vi "CameraSend Images To PC Loop.vi"(8 "error in (no error)":errorcluster, 11 "CameraDevRef":T1) -> ()   [LabVIEW 2014]
doc: "This VI is used to send images to the dashboard using the second enet port on the 8 slot controller. This is provided for compatibility, but is higher overhead than using the Camera MJPG approach.\n\nThis software is licensed. Open the labview\\readme\\WPI Robotics Library Open Source License.txt file for more information."
uses:
  <vilib>/Rock Robotics/WPI/Camera/WPI_CameraDevRef.ctl
  typedefs/vision/vision enable.ctl
  <vilib>/Rock Robotics/SystemInterfaces/NetworkCommunication/NetComm_UsageReport_ResourceType.ctl
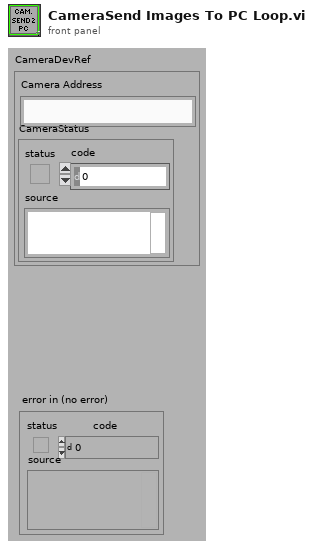
[diagram p1: front panel]
types:
  T1 = typedef "WPI_CameraDevRef.ctl" = cluster{"Camera Address":string, "CameraStatus":errorcluster}
  T2 = typedef "vision enable.ctl" = enum16{"Enable", "Disable", "Stop"}
  T3 = cluster{"fps":i32, "compression":i32, "compression 2":i32}
  T4 = typedef "NetComm_UsageReport_ResourceType.ctl" = enum8{"Controller", "Module", "Language", "CANPlugin", "Accelerometer", "ADXL345", "AnalogChannel", "AnalogTrigger", "AnalogTriggerOutput", "CANJaguar", "Compressor", "Counter", "Dashboard", "DigitalInput", "DigitalOutput", "DriverStationCIO", "DriverStationEIO", "DriverStationLCD", "Encoder", "GearTooth", "Gyro", "I2C", "Framework", "Jaguar", "Joystick", "Kinect", "KinectStick", "PIDController", "Preferences", "PWM", "Relay", "RobotDrive", "SerialPort", "Servo", "Solenoid", "SPI", "Task", "Ultrasonic", "Victor", "Button", "Command", "AxisCamera", "PCVideoServer", "SmartDashboard", "Talon", "HiTechnicColorSensor", "HiTechnicAccel", "HiTechnicCompass", "SRF08", "AnalogOutput", "Victor SP", "Talon SRX", "CAN Talon SRX"}
  T5 = enum16{"Update Mode", "Get Image", "Get Image Data"}
  T6 = typedef "Image Type" = u32
  T7 = typedef "IMAQ Image.ctl" = refnum<image>
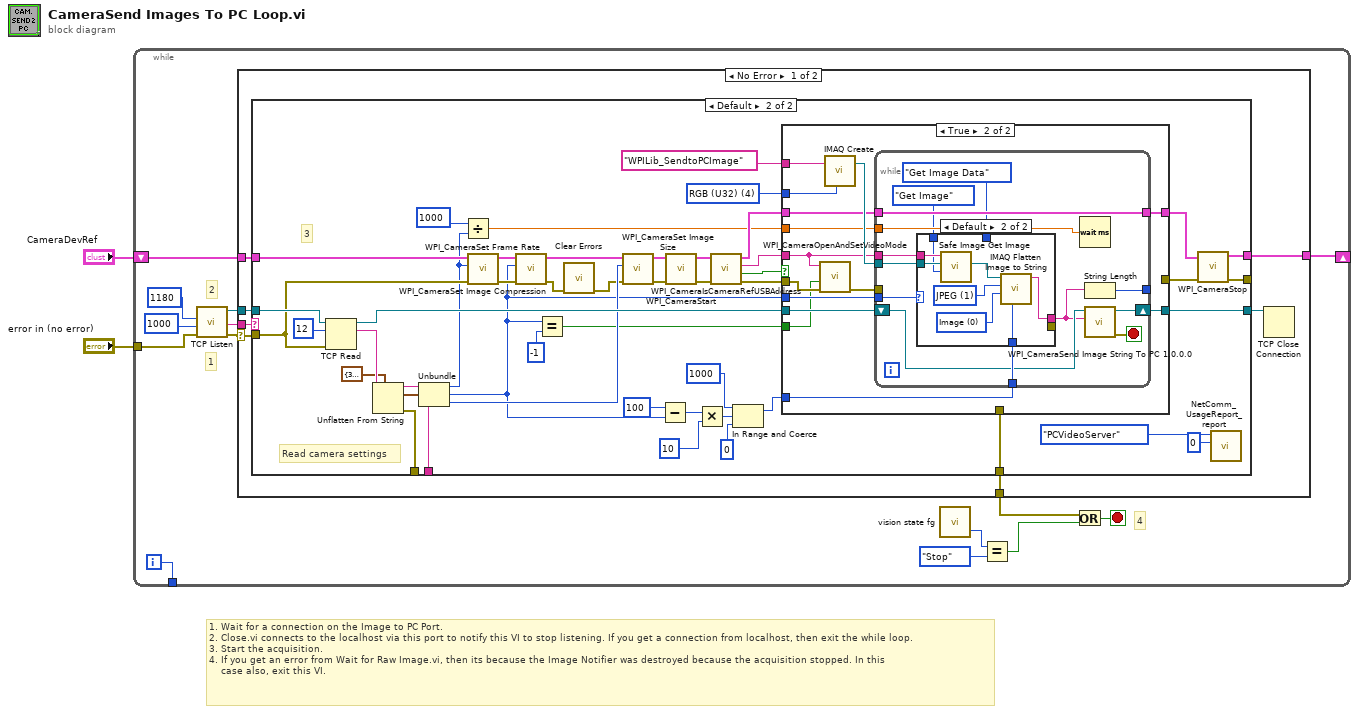
[diagram p0: block diagram]
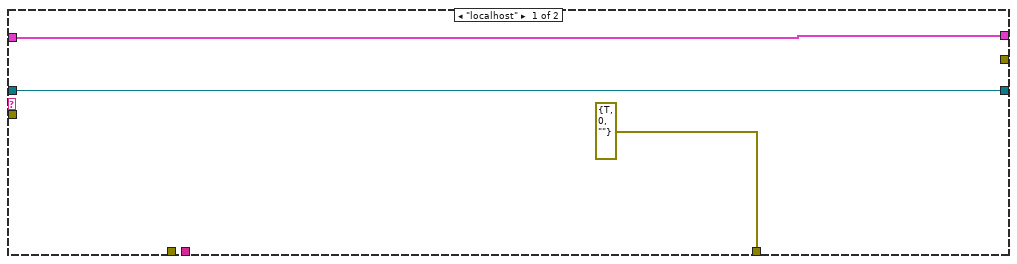
[diagram p2: hidden frame]
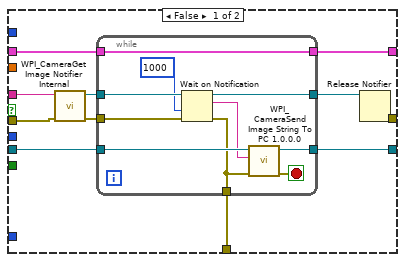
[diagram p3: hidden frame]
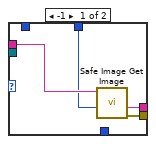
[diagram p4: hidden frame]
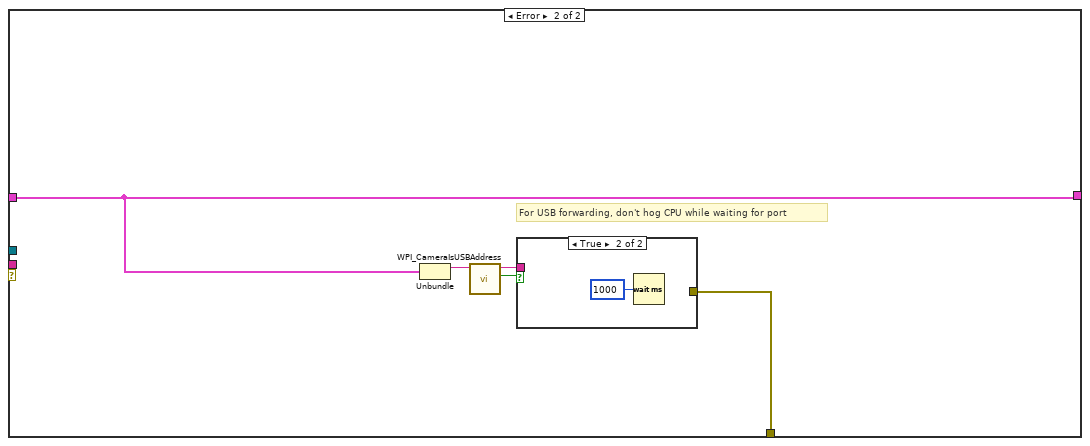
[diagram p5: hidden frame]
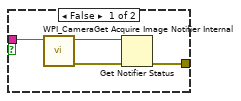
[diagram p6: hidden frame]
diagram:
  # "1. Wait for a connection on the Image to PC Port.\n2. Close.vi connects to the localhost via this port to notify this VI to stop listening. If you get a connection from localhost, then exit the while loop.\n3. Start the acquisition.\n4. If you get an error from Wait for Raw Image.vi, then its because the Image Notifier was destroyed because the acquisition stopped. In this\n    case also, exit this VI."
  n1 = while {
    tunnel: "error in (no error)" -> [w13]
    shift-right: [w16] -> _
    shift-left: "CameraDevRef" -> [w14]
    tunnel: [w8] -> _
    i -> [w8]
    stop <- w5 stop-if-true
    # "4"
    # "1"
    # "2"
    n2 = call <vilib>:"TCP Listen.vi"("error in (no error)"=w13, "timeout ms (wait forever: -1)"=u16 1000 ("port"), "port"=u16 1180) -> ("error out"=w10:errorcluster, "remote address"=w15:string, "connection ID"=w12:refnum<k5>)  [unwired: 1 in, 5 out]
    n3 = case shown="No Error" w10 {
      selector: w10 -> [w17 _]
      tunnel: [w23 w137] -> w16
      tunnel: w15 -> [w22 _]
      tunnel: w14 -> [w21 w137]
      tunnel: w12 -> [w20 _]
      tunnel: [w19 w138] -> w4
      frame No Error {
        n4 = case shown="Default" w22 {
          tunnel: [w26 w71] -> w23
          tunnel: w21 -> [w26 w53]
          tunnel: w17 -> [_ w49]
          tunnel: w20 -> [w24 w57]
          tunnel: [errorcluster {"status"=TRUE, "code"=0, "source"=""} ("error out 2") w73] -> w19
          tunnel: [w24 w72] -> w18
          tunnel: [_ w70] -> _
          tunnel: [_ w28] -> _
          tunnel: [_ w27] -> _
          frame "localhost" {
          }
          frame Default {
            w64 = T6 4 items=["Grayscale (U8)", "Grayscale (I16)", "Grayscale (SGL)", "Complex (CSG)", "RGB (U32)", "HSL (U32)", "RGB (U64)", "Grayscale (U16)"] ("Image Type")
            # "Read camera settings"
            # "3"
            n5 = TCP Read(connection ID=w57, bytes to read=12, error in (no error)=w49) -> (connection ID out=w56:refnum<k5>, data out=w54:string)  [unwired: 2 in, 1 out]
            n6 = Unflatten From String(type=T3 {"fps"=30, "compression"=32, "compression 2"=32} ("Camera Settings"), binary string=w54) -> (rest of the binary string=w27:string, value=w46:T3, error out=w28:errorcluster)  [unwired: 3 in]
            n7 = Unbundle(w46) -> ("fps"=w43:i32, "compression"=w32:i32, "compression 2"=w45:i32)
            n8 = Divide(x=u16 1000 ("port"), y=w43) -> (x/y=w42:dbl)
            n9 = call <vilib>:"WPI_CameraSet Frame Rate.vi"("error in (no error)"=w49, "Frame Rate (fps)"=w43, "CameraDevRef"=w53) -> ("error out"=w48:errorcluster, "CameraDevRef Out"=w52:T1)  [unwired: 7 in]
            n10 = call <vilib>:"WPI_CameraSet Image Compression.vi"("error in (no error)"=w48, "Compression"=w32, "CameraDevRef"=w52) -> ("error out"=w30:errorcluster, "CameraDevRef Out"=w51:T1)  [unwired: 7 in]
            n11 = Equal?(x=w32, y=-1) -> (x = y?=w31:bool)
            n12 = call <vilib>:"Clear Errors.vi"("error in (no error)"=w30) -> ("error out"=w29:errorcluster)  [unwired: 5 in, 1 out]
            n13 = call <vilib>:"WPI_CameraSet Image Size.vi"("error in (no error)"=w29, "Image Size"=w45, "CameraDevRef"=w51) -> ("error out"=w47:errorcluster, "CameraDevRef Out"=w50:T1)  [unwired: 7 in]
            n14 = Subtract(x=100, y=w32) -> (x-y=w37:i32)
            n15 = call <vilib>:"WPI_CameraStart.vi"("error in (no error)"=w47, "CameraDevRef"=w50) -> ("error out"=w61:errorcluster, "CameraDevRef Out"=w59:T1)  [unwired: 8 out]
            n16 = Multiply(x=w37, y=10) -> (x*y=w39:i32)
            n17 = call <vilib>:"WPI_CameraIsCameraRefUSBAddress.vi"("error in (no error)"=w61, "CameraDevRef"=w59) -> ("error out"=w60:errorcluster, "USB?"=w62:bool, "Camera Address Out"=w63:string, "CameraDevRef out"=w58:T1)  [unwired: 6 in]
            n18 = In Range and Coerce(upper limit=1000, x=w39, lower limit=0) -> (coerced(x)=w35:i32)  [unwired: 1 out]
            n19 = case shown="True" w62 {
              tunnel: w56 -> [w84 w108]
              tunnel: [w83 _] -> w73
              tunnel: [w82 w107] -> w72
              tunnel: w60 -> [w81 w98]
              tunnel: w63 -> [w79 w97]
              tunnel: [w78 w102] -> w69
              tunnel: w58 -> [w77 w103]
              tunnel: [w75 _] -> w68
              tunnel: "WPILib_SendtoPCImage" -> [_ w105]
              tunnel: w64 -> [_ w104]
              tunnel: w35 -> [_ w101]
              tunnel: w42 -> [_ w100]
              tunnel: w32 -> [_ w99]
              tunnel: w31 -> [_ w95]
              frame False {
                n20 = call <vilib>:"WPI_CameraGet Image Notifier Internal.vi"("error in (no error)"=w81, "Camera Address"=w79) -> ("error out"=w80:errorcluster, "Image Notifier"=w76:refnum<notifier>)  [unwired: 8 out]
                n21 = while {
                  tunnel: w80 -> [w90]
                  tunnel: w84 -> [w94]
                  tunnel: [w87] -> w83
                  tunnel: [w92] -> w82
                  tunnel: [w91] -> w78
                  tunnel: w77 -> [w91]
                  tunnel: w76 -> [w89]
                  tunnel: [w85] -> w74
                  stop <- w93 stop-if-true
                  n22 = Wait on Notification(notifier=w89, timeout in ms (-1)=1000 ("Timeout in ms (-1)"), error in (no error)=w90) -> (notifier out=w85:refnum<notifier>, notification=w88:string, error out=w87:errorcluster)  [unwired: 2 out]
                  n23 = call <vilib>:"WPI_CameraSend Image String To PC 1.0.0.0.vi"("error in (no error)"=w87, "String"=w88, "TCP Connection ID"=w94) -> ("error out"=w93:errorcluster, "TCP Connection ID out"=w92:refnum<k5>)  [unwired: 7 out]
                }
                n24 = Release Notifier(notifier=w74) -> (error out=w75:errorcluster)  [unwired: 1 in, 3 out]
              }
              frame True {
                n25 = call <vilib>:"WPI_CameraOpenAndSetVideoMode.vi"("error in (no error)"=w98, "USB JPEG"=w95, "Camera Address Out"=w97) -> ("error out"=w96:errorcluster)  [unwired: 8 in]
                n26 = call "IMAQ Create"("Image Name"=w105, "Image Type"=w104) -> ("New Image"=w106:T7)  [unwired: 3 in, 1 out]
                n27 = while {
                  tunnel: w97 -> [w120]
                  shift-right: [w121] -> w107
                  shift-left: w108 -> [w114]
                  tunnel: w106 -> [w119]
                  tunnel: [w117] -> w102
                  tunnel: w103 -> [w117]
                  tunnel: w101 -> [w116]
                  tunnel: w100 -> [w115]
                  tunnel: [w112] -> _
                  tunnel: w99 -> [w111]
                  tunnel: w96 -> [_]
                  stop <- w118 stop-if-true
                  n28 = case shown="Default" w111 {
                    tunnel: [w124 w133] -> w113
                    tunnel: w120 -> [w125 w129]
                    tunnel: w119 -> [_ w128]
                    tunnel: w116 -> [_ w130]
                    tunnel: [w123 _] -> _
                    tunnel: T5."Get Image Data" ("Operation") -> [w122 _]
                    tunnel: T5."Get Image" ("Operation") -> [_ w126]
                    frame -1 {
                      n29 = call <vilib>:"Safe Image Get Image.vi"("Operation"=w122, "Session In"=w125) -> ("error out"=w123:errorcluster, "Image Data String"=w124:string)  [unwired: 6 in, 2 out]
                    }
                    frame Default {
                      w131 = 0 items=["Image", "Image and Vision Info", "Reference to Image"] ("Type of Flatten (Image and Vision Info)")
                      w132 = 1 items=["None", "JPEG", "PACKED BINARY"] ("Compression (None)")
                      n30 = call <vilib>:"Safe Image Get Image.vi"("Operation"=w126, "Image In"=w128, "Session In"=w129) -> ("Image Out"=w127:T7)  [unwired: 5 in, 3 out]
                      n31 = call "IMAQ Flatten Image to String"("Quality (750)"=w130, "Type of Flatten (Image and Vision Info)"=w131, "Compression (None)"=w132, "Image"=w127) -> ("Data String"=w133:string)  [unwired: 6 in, 1 out]
                    }
                  }
                  n32 = Wait (ms)(milliseconds to wait=w115) -> ()  [unwired: 1 out]
                  n33 = String Length(string=w113) -> (length=w112:i32)
                  n34 = call <vilib>:"WPI_CameraSend Image String To PC 1.0.0.0.vi"("String"=w113, "TCP Connection ID"=w114) -> ("error out"=w118:errorcluster, "TCP Connection ID out"=w121:refnum<k5>)  [unwired: 1 in, 7 out]
                }
              }
            }
            n35 = call <vilib>:"WPI_CameraStop.vi"("error in (no error)"=w68, "CameraDevRef"=w69) -> ("error out"=w70:errorcluster, "CameraDevRef Out"=w71:T1)  [unwired: 8 out]
            n36 = call <vilib>:"NetComm_UsageReport_report.vi"("Instance Number"=u8 0, "Resource Type"=NetComm_UsageReport_ResourceType."PCVideoServer") -> ()  [unwired: 10 in]
          }
        }
        n37 = TCP Close Connection(connection ID=w18) -> ()  [unwired: 1 in, 3 out]
      }
      frame Error {
        # "For USB forwarding, don't hog CPU while waiting for port"
        n38 = Unbundle(w137) -> ("Camera Address"=w136:string)  [unwired: 1 out]
        n39 = call <vilib>:"WPI_CameraIsUSBAddress.vi"("Camera Address In"=w136) -> ("USB?"=w134:bool, "Camera Address Out"=w135:string)  [unwired: 8 in, 1 out]
        n40 = case shown="True" w134 {
          tunnel: [w142 _] -> w138
          tunnel: w135 -> [w139 _]
          frame False {
            n41 = call <vilib>:"WPI_CameraGet Acquire Image Notifier Internal.vi"("Camera Address"=w139) -> ("error out"=w140:errorcluster, "Acquire Image Notifier"=w141:refnum<notifier>)  [unwired: 1 in, 8 out]
            n42 = Get Notifier Status(notifier=w141, error in (no error)=w140) -> (error out=w142:errorcluster)  [unwired: 4 out]
          }
          frame True {
            n43 = Wait (ms)(milliseconds to wait=u32 1000) -> ()  [unwired: 1 out]
          }
        }
      }
    }
    n44 = call "vision state fg.vi"() -> ("State Out"=w7:T2)  [unwired: 2 in, 1 out]
    n45 = Equal?(x=w7, y=vision_enable."Stop") -> (x = y?=w3:bool)
    n46 = Or(x=w4, y=w3) -> (x .or. y?=w5:bool)
  }
